vi "RichToFlatnixnet_grpc_FlexRayCommResponse.vi"(5 "OutputClusterType":T1, 11 "InputCluster":T3) -> (3 "OutputCluster":T1)   [LabVIEW 2025, in "grpc-xnet_client.lvlib"]
uses:
  nixnet_grpc_FlexRayCommResponse.ctl
  nixnet_grpc_FlexRayPocState.ctl
  nixnet_grpc_FlexRayCommResponse_Flat.ctl
  grpc-xnet_client.lvlib
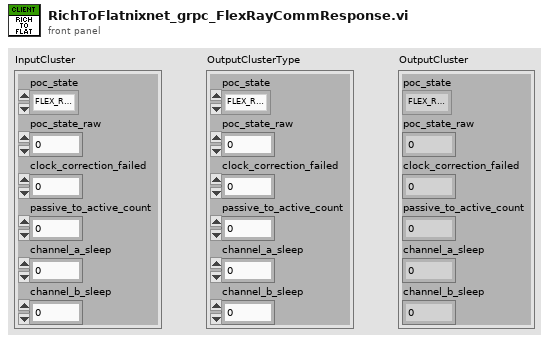
[diagram p1: front panel]
types:
  T1 = typedef "grpc-xnet_client.lvlib/nixnet_grpc_FlexRayCommResponse_Flat.ctl" = cluster{"poc_state":T2, "poc_state_raw":u32, "clock_correction_failed":u32, "passive_to_active_count":u32, "channel_a_sleep":u32, "channel_b_sleep":u32}
  T2 = typedef "grpc-xnet_client.lvlib/nixnet_grpc_FlexRayPocState.ctl" = enum32{"FLEX_RAY_POC_STATE_DEFAULT_CONFIG", "FLEX_RAY_POC_STATE_READY", "FLEX_RAY_POC_STATE_NORMAL_ACTIVE", "FLEX_RAY_POC_STATE_NORMAL_PASSIVE", "FLEX_RAY_POC_STATE_HALT", "FLEX_RAY_POC_STATE_MONITOR", "FLEX_RAY_POC_STATE_CONFIG"}
  T3 = typedef "grpc-xnet_client.lvlib/nixnet_grpc_FlexRayCommResponse.ctl" = cluster{"poc_state":T2, "poc_state_raw":u32, "clock_correction_failed":u32, "passive_to_active_count":u32, "channel_a_sleep":u32, "channel_b_sleep":u32}
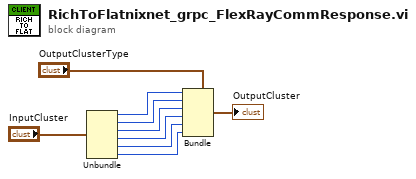
[diagram p0: block diagram]
diagram:
  n1 = Unbundle "Unbundle"("InputCluster") -> ("poc_state"=w6:T2, "poc_state_raw"=w5:u32, "clock_correction_failed"=w4:u32, "passive_to_active_count"=w3:u32, "channel_a_sleep"=w2:u32, "channel_b_sleep"=w1:u32)
  n2 = Bundle "Bundle"(cluster="OutputClusterType", "poc_state"=w6, "poc_state_raw"=w5, "clock_correction_failed"=w4, "passive_to_active_count"=w3, "channel_a_sleep"=w2, "channel_b_sleep"=w1) -> (→"OutputCluster":T1)
